vi "example.vi"() -> ()   [LabVIEW 2014]
uses:
  TelnetOperations.ctl
panel:
  out "NeedRestart?":bool
  in  "address":string="192.168.1.2"
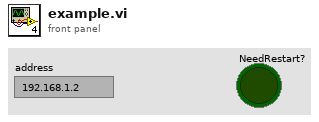
[diagram p1: front panel]
types:
  T1 = typedef "TelnetOperations.ctl" = enum16{"Open", "Write", "Read", "Start", "Restart", "Stop", "VerifyProcess", "Close"}
  T2 = typedef "Telnet Session.ctl" = refnum<k1>
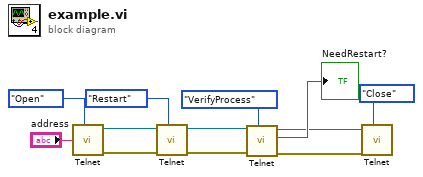
[diagram p0: block diagram]
diagram:
  n1 = call "Telnet.vi"("operaiton"=TelnetOperations."Open", "address"="address") -> ("error out"=w8:errorcluster, "telnet connection out"=w10:T2)  [unwired: 6 in, 2 out]
  n2 = call "Telnet.vi"("operaiton"=TelnetOperations."Restart", "error in (no error)"=w8, "telnet connection in"=w10) -> ("error out"=w7:errorcluster, "telnet connection out"=w4:T2)  [unwired: 5 in, 2 out]
  n3 = call "Telnet.vi"("operaiton"=TelnetOperations."VerifyProcess", "error in (no error)"=w7, "telnet connection in"=w4) -> ("error out"=w2:errorcluster, "NeedRestart?"=→"NeedRestart?":bool, "telnet connection out"=w3:T2)  [unwired: 5 in, 1 out]
  n4 = call "Telnet.vi"("operaiton"=TelnetOperations."Close", "error in (no error)"=w2, "telnet connection in"=w3) -> ()  [unwired: 5 in, 4 out]
